vi "1.vi"() -> ()   [LabVIEW 2020]
uses:
  <vilib>/numeric/Random Number (Range) U64.vi
  bf688a23-0469-42af-9409-3477dd1fc06d.vi
  e0c3b0d3-6cb3-46d4-9eec-1810efa34836.vi
  <vilib>/numeric/sub_Random U32.vi
  <vilib>/Comparison/Less/Less Functor/Less Functor.lvclass
  <vilib>/Comparison/Equal/Equal Functor/Equal Functor.lvclass
panel:
  out "Array":u64[](array[numeric])
  out "Index":i32[](array[numeric])
  out "sorted array":u64[](array[numeric])
  out "Max 3 elements":u64[](array[numeric])
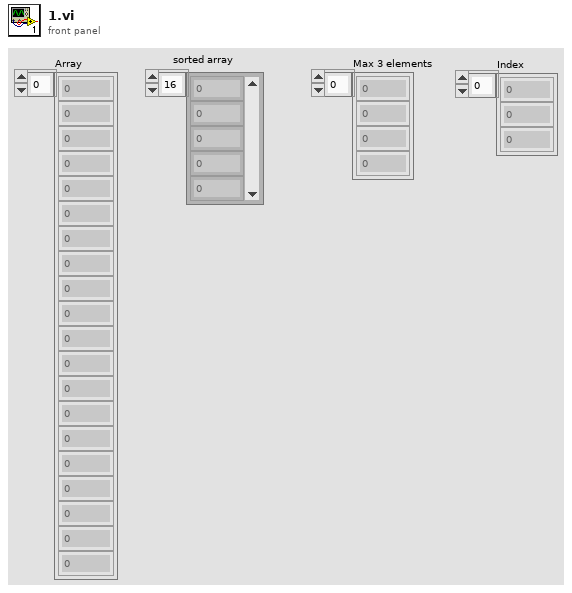
[diagram p1: front panel]
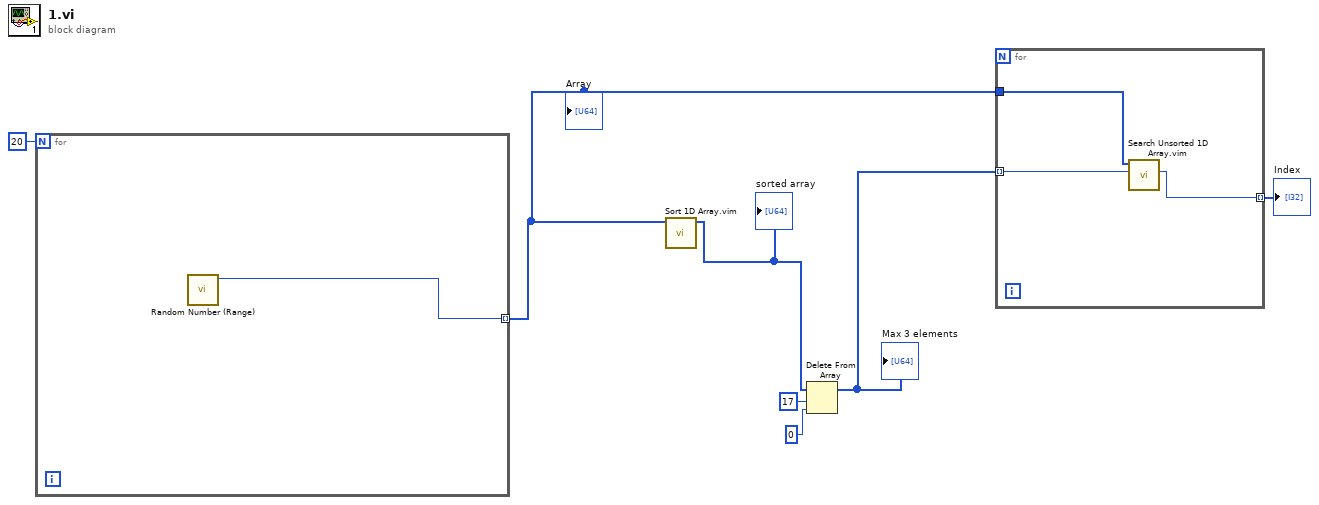
[diagram p0: block diagram]
diagram:
  n1 = for {
    N: 20 -> [_]
    tunnel: [w8] -> w3 mode=indexing
    n2 = call-poly <vilib>:"Random Number (Range).vi"() -> ("number"=w8:u64)  [unwired: 11 in]
  }
  "Array" <- w3
  n3 = call "Sort 1D Array.vim"("unsorted array"=w3) -> ("sorted array"=w4:u64[])  [unwired: 10 in]
  "sorted array" <- w4
  n4 = Delete From Array(array=w4, length=17, index=0) -> (array with subset deleted=w2:u64[])  [unwired: 1 out]
  "Max 3 elements" <- w2
  n5 = for {
    tunnel: w3 -> [w11]
    tunnel: w2 -> [w10] mode=indexing
    tunnel: [w9] -> w1 mode=indexing
    n6 = call "Search Unsorted 1D Array.vim"("element"=w10, "unsorted 1D array"=w11) -> ("index of element"=w9:i32)  [unwired: 9 in]
  }
  "Index" <- w1
